vi "Step2_BandPass_AntiHarmonic.vi"(9 "s_axis_data_tdata":fxp<+/-,32,30>, 10 "s_axis_data_tvalid":bool) -> (1 "m_axis_data_tdata":fxp<+/-,48,48>, 2 "m_axis_data_tvalid":bool, 3 "s_axis_data_tready":bool)   [LabVIEW 2018]
uses:
  <vilib>/rvi/XilinxIP/XIPIN_XNode/niFpgaXIPIN.xnode
  Deprecated_Delete/DigitalFilterDesign/FIR_Filter_Configuration/FIR Compiler/xsim.dir/FIR_Compiler_3CE652926F5B43F18022D1349C670FA0/xsimk_3CE652926F5B43F18022D1349C670FA0.dll
  <vilib>/rvi/IPIntegrationNode/IPINode_Xnode/niFpgaIPINode.xnode
  <vilib>/rvi/IPIntegrationNode/IPINode_Typedef/niFpgaIPINodeSupportedFamilies.ctl
  <vilib>/rvi/IPIntegrationNode/IPINode_Utilities/niFpgaIPINodeSimCore.vi
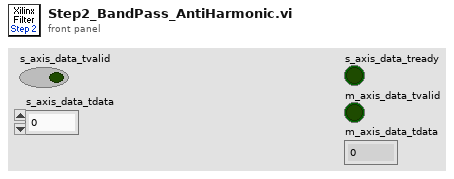
[diagram p1: front panel]
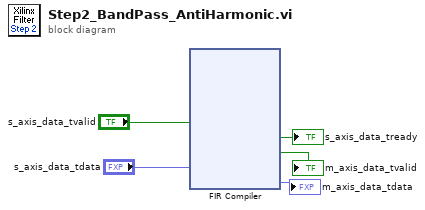
[diagram p0: block diagram]
diagram:
  n1 = xnode ("FIR Compiler")("s_axis_data_tvalid"="s_axis_data_tvalid", "s_axis_data_tdata"="s_axis_data_tdata") -> ("s_axis_data_tready"=→"s_axis_data_tready":bool, "m_axis_data_tvalid"=→"m_axis_data_tvalid":bool, "m_axis_data_tdata"=→"m_axis_data_tdata":fxp<+/-,48,48>)
